vi "ABAPI Dist Get File Base Name.vi"(2 "new extension":string, 3 "file name":string) -> (0 "new name":string, 1 "base name":string)   [LabVIEW 2020]
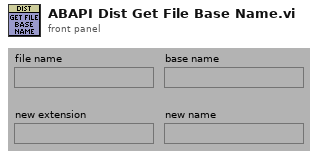
[diagram p1: front panel]
types:
  T1 = enum32{"invalid OS target", "Mac OS", "Windows 3.1", "Windows 95/NT", "Solaris 1", "Solaris 2", "HP-UX", "PowerMAX", "Linux", "Irix", "Rhapsody", "BeOS", "AIX", "OSF1", "VxWorks", "PharLap", "Carbon", "RTX", "Windows x64", "Linux x64", "Mac OS X x64"}
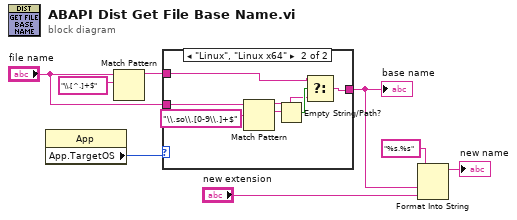
[diagram p0: block diagram]
diagram:
  n1 = property class="App"() -> ("App.TargetOS"=w2:T1)  [unwired: 2 in, 2 out]
  n2 = Match Pattern(string="file name", regular expression="\\.[^.]+$") -> (before substring=w7:string)  [unwired: 1 in, 3 out]
  n3 = case shown="\"Linux\", \"Linux x64\"" w2 {
    tunnel: [w9 w10] -> w3
    tunnel: w7 -> [w9 w12]
    tunnel: "file name" -> [_ w15]
    frame Default {
    }
    frame "Linux", "Linux x64" {
      n4 = Match Pattern(string=w15, regular expression="\\.so\\.[0-9\\.]+$") -> (before substring=w11:string, match substring=w14:string)  [unwired: 1 in, 2 out]
      n5 = Empty String/Path?(string/path=w14) -> (empty?=w13:bool)
      n6 = Select(t=w12, s=w13, f=w11) -> (s? t:f=w10:string)
    }
  }
  "base name" <- w3
  n7 = Format Into String(format string="%s.%s" ("Format String"), w3, "new extension") -> (resulting string=→"new name":string)  [unwired: 2 in, 1 out]
